vi "ModBus test.vi"() -> ()   [LabVIEW 2020]
uses:
  <vilib>/Modbus/master/Create Master Instance (TCP).vi
  <vilib>/Modbus/master/Modbus Master.lvclass
panel:
  out "coils":bool[](array[boolean])
  in  "coil to write":bool
  in  "starting coil address":u16
  out "*(type *) &x":string
  out "register values":u16[](array[numeric])=[18537, 8308, 26725, 29285, 8224, 8224, 8224, 8224, 8224, 8224, 8224, 8224, 8224, 8224, 8224, 8224, 8224, 8224, 8224, 8224, 8224, 8224, 8224, 8224, 8224, 8224, 8224, 8224, 8224, 8224, 8224, 8224, 8224, 8224, 8224, 8224, 8224, 8224, 8224, 8224, 8224, 8224, 8224, 8224, 8224, 8224, 8224, 8224, 8224, 8224, 8224, 8224, 8224, 8224, 8224, 8224, 8224, 8224, 8224, 8224, 8224, 8224, 8224, 8224, 8224, 8224, 0, 0, 0, 0, 0, 0, 0, 0, 0, 0, 0, 0, 0, 0, 0, 0, 0, 0, 0, 0, 0, 0, 0, 0, 0, 0, 0, 0, 0, 0, 0, 0, 0, 0, 0, 0, 0, 0, 0, 0, 0, 0, 0, 0, 0, 0, 0, 0, 0, 0, 0, 0, 0, 0, 0, 0, 0, 0, 0]
  in  "number of inputs":u16=125
  in  "starting holding address":u16=1200
  in  "address":string="172.22.117.193"
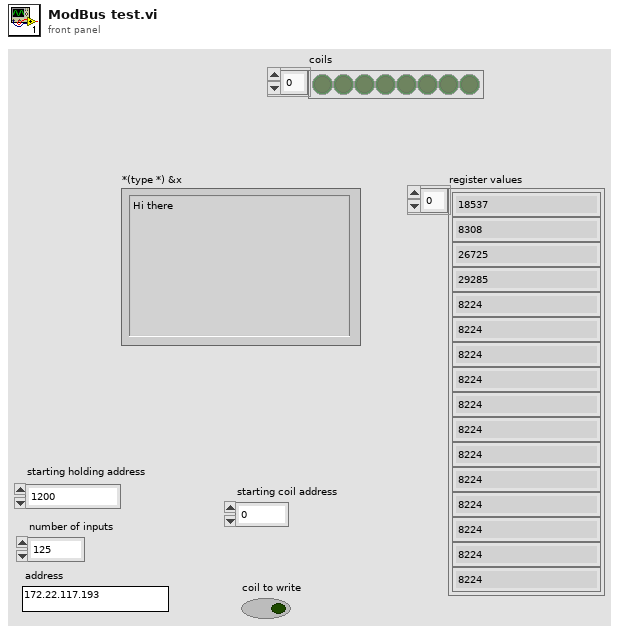
[diagram p1: front panel]
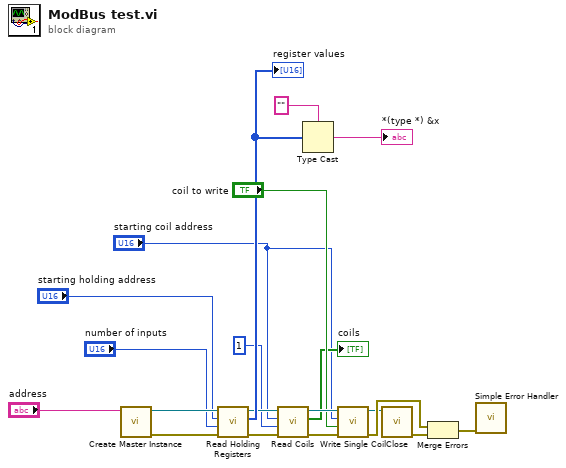
[diagram p0: block diagram]
diagram:
  n1 = call-poly <vilib>:"Create Master Instance.vi"("address"="address") -> ("error out"=w19:errorcluster, "TCP master instance"=w20:refnum<class "Modbus Master.lvclass">)  [unwired: 9 in]
  n2 = call-dynamic "Read Holding Registers.vi"("error in (no error)"=w19, "number of holding registers"="number of inputs", "starting address"="starting holding address", "Modbus master in"=w20) -> ("error out"=w17:errorcluster, "register values"=w15:u16[], "Modbus master out"=w11:refnum<class "Modbus Master.lvclass">)  [unwired: 5 in]
  "register values" <- w15
  n3 = call-dynamic "Read Coils.vi"("error in (no error)"=w17, "number of coils"=u16 1 ("number of inputs"), "starting address"="starting coil address", "Modbus master in"=w11) -> ("error out"=w12:errorcluster, "coil values"=→"coils":bool[], "Modbus master out"=w9:refnum<class "Modbus Master.lvclass">)  [unwired: 5 in]
  n4 = Type Cast(type="", x=w15) -> (*(type *) &x=→"*(type *) &x":string)
  n5 = call-dynamic "Write Single Coil.vi"("error in (no error)"=w12, "coil value"="coil to write", "address"="starting coil address", "Modbus master in"=w9) -> ("error out"=w10:errorcluster, "Modbus master out"=w8:refnum<class "Modbus Master.lvclass">)  [unwired: 6 in]
  n6 = call-dynamic "Close.vi"("Modbus master in"=w8) -> ("error out"=w18:errorcluster)  [unwired: 10 in]
  n7 = Merge Errors(w10, w18) -> (w16:errorcluster)
  n8 = call <vilib>:"Simple Error Handler.vi"("error in (no error)"=w16) -> ()  [unwired: 4 in, 5 out]
